vi "VPA QC Calc Values.vi"(9 "Y in":dbl[](array[numeric]), 10 "X in":dbl[](array[numeric]), 11 "Array in":cluster{"X":dbl[], "Y":dbl[]}[](array[cluster])) -> (1 "intercept":dbl, 2 "X out":dbl[](array[numeric]), 3 "slope":dbl format="%.5g", 4 "Y out":dbl[](array[numeric]), 5 "Array out":cluster{"X":dbl[], "Y":dbl[]}[](array[cluster]), 6 "Suggested Volts":dbl)   [LabVIEW 2013]
uses:
  <vilib>/ptbypt/NI_PtbyPt.lvlib
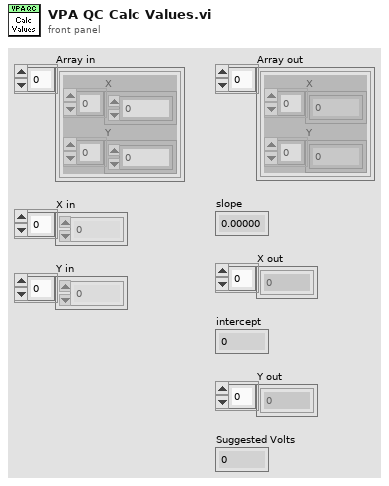
[diagram p1: front panel]
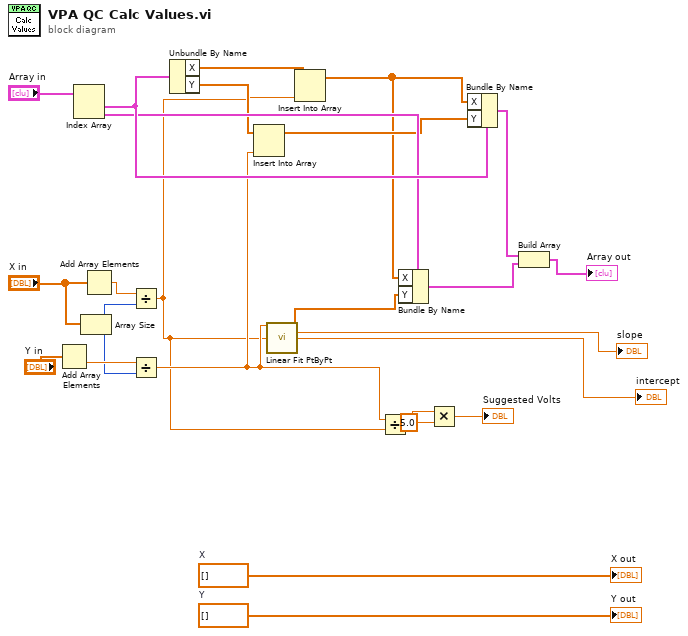
[diagram p0: block diagram]
diagram:
  w15 = dbl[] []  # X
  w16 = dbl[] []  # Y
  n1 = Add Array Elements(numeric array="Y in") -> (sum=w11:dbl)
  n2 = Index Array(array="Array in") -> (element #1=w8:cluster{"X":dbl[], "Y":dbl[]}, element #2=w7:cluster{"X":dbl[], "Y":dbl[]})  [unwired: 2 in]
  n3 = Array Size(array="X in") -> (size(s)=w9:i32)
  n4 = Add Array Elements(numeric array="X in") -> (sum=w10:dbl)
  n5 = Divide(x=w10, y=w9) -> (x/y=w1:dbl)
  n6 = Divide(x=w11, y=w9) -> (x/y=w4:dbl)
  n7 = Unbundle By Name(w8) -> ("X"=w6:dbl[], "Y"=w5:dbl[])
  n8 = Insert Into Array(array=w5, new element=w4) -> (w3:dbl[])  [unwired: 1 in]
  n9 = call <vilib>:"Linear Fit PtByPt.vi"("y"=w4, "x"=w1) -> ("Best Linear Fit"=w22:dbl[], "slope"=→"slope":dbl, "intercept"=→"intercept":dbl)  [unwired: 9 in, 2 out]
  n10 = Insert Into Array(array=w6, new element=w1) -> (w2:dbl[])  [unwired: 1 in]
  n11 = Divide(x=w4, y=w1) -> (x/y=w12:dbl)
  n12 = Bundle By Name(cluster=w7, "X"=w2, "Y"=w22) -> (w23:cluster{"X":dbl[], "Y":dbl[]})
  n13 = Multiply(x=w12, y=5.0) -> (x*y=→"Suggested Volts":dbl)
  n14 = Bundle By Name(cluster=w8, "X"=w2, "Y"=w3) -> (w19:cluster{"X":dbl[], "Y":dbl[]})
  n15 = Build Array(w19, w23) -> (→"Array out":cluster{"X":dbl[], "Y":dbl[]}[])
  "Y out" <- w16
  "X out" <- w15
